vi "Split and Invert u32 to two u16.vi"(9 "Data Invert [F]":bool, 10 "Input (u32)":u32) -> (1 "LSB (u16)":u16, 2 "MSB (u16)":u16)   [LabVIEW 2015]
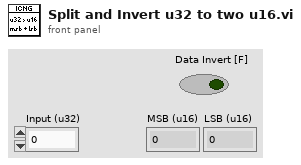
[diagram p1: front panel]
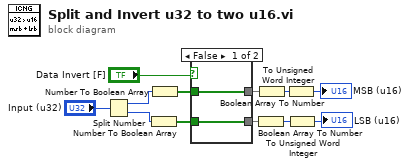
[diagram p0: block diagram]
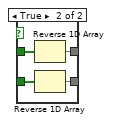
[diagram p2: hidden frame]
diagram:
  n1 = Split Number(x="Input (u32)") -> (hi(x)=w8:u16, lo(x)=w7:u16)
  n2 = Number To Boolean Array(number=w7) -> (Boolean array=w12:bool[])
  n3 = Number To Boolean Array(number=w8) -> (Boolean array=w10:bool[])
  n4 = case shown="False" "Data Invert [F]" {
    tunnel: w12 -> [w13 w18]
    tunnel: [w13 w17] -> w11
    tunnel: w10 -> [w14 w16]
    tunnel: [w14 w15] -> w9
    frame False {
    }
    frame True {
      n5 = Reverse 1D Array(array=w16) -> (reversed array=w15:bool[])
      n6 = Reverse 1D Array(array=w18) -> (reversed array=w17:bool[])
    }
  }
  n7 = Boolean Array To Number(Boolean array=w11) -> (number=w4:u32)
  n8 = Boolean Array To Number(Boolean array=w9) -> (number=w5:u32)
  n9 = To Unsigned Word Integer(number=w5) -> (unsigned 16bit integer=→"MSB (u16)":u16)
  n10 = To Unsigned Word Integer(number=w4) -> (unsigned 16bit integer=→"LSB (u16)":u16)
